vi "CLD 16 solution.vi"() -> ()   [LabVIEW 2020]
doc: "CLD 16 Exercise"
uses:
  Controls/CLD 16 Control Panel.ctl
  Controls/CLD 16 Status Panel.ctl
panel:
  in  "Stop Button":bool
  out "Line Two Active":bool
  out "Line One Active":bool
  in  "Control Panel Two":T1 {"Tons of Peanuts" scale=0.0..10.0}
  out "Process Control":T2 {"Process Value" format="%#.3g"}
  in  "Control Panel One":T1 {"Tons of Peanuts" scale=0.0..10.0}
  # "Display Panel"
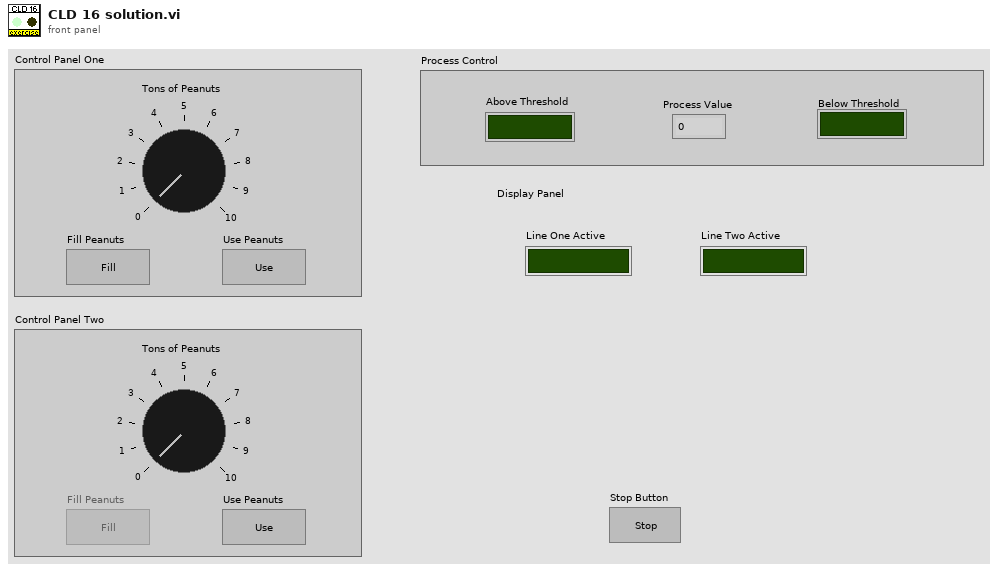
[diagram p1: front panel]
types:
  T1 = typedef "CLD 16 Control Panel.ctl" = cluster{"Tons of Peanuts":i8, "Fill Peanuts":bool, "Use Peanuts":bool}
  T2 = typedef "CLD 16 Status Panel.ctl" = cluster{"Above Threshold":bool, "Below Threshold":bool, "Process Value":dbl}
  T3 = enum8{"Enabled", "Disabled", "Disabled and Grayed Out"}
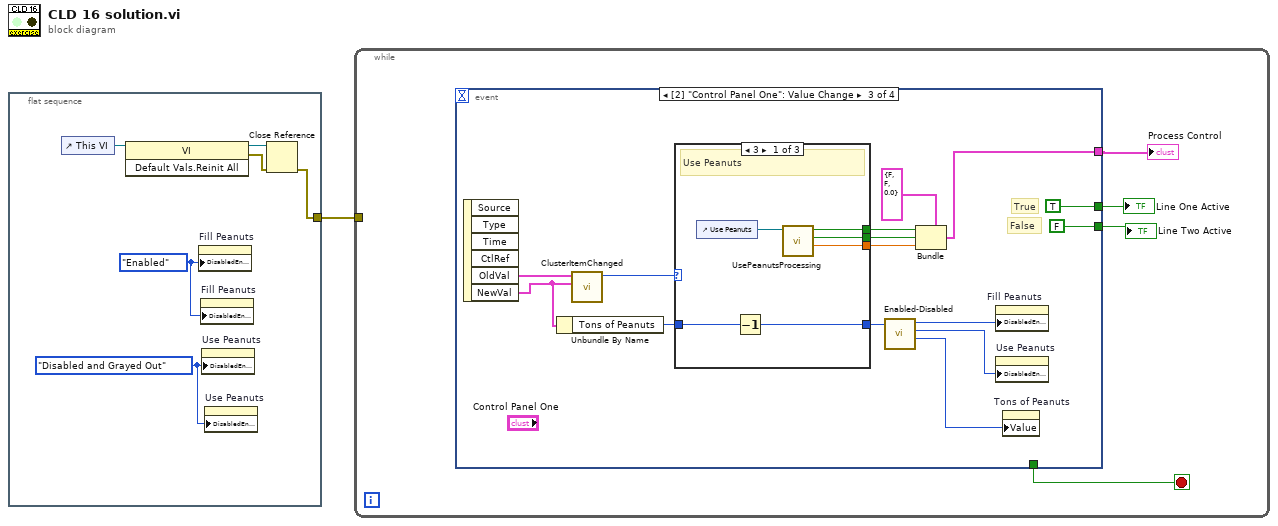
[diagram p0: block diagram]
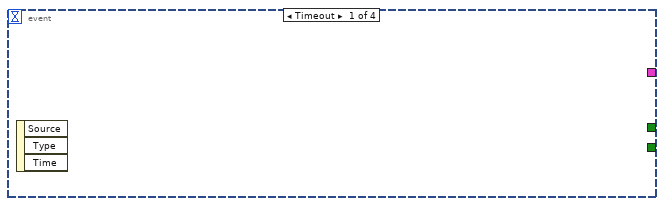
[diagram p2: hidden frame]
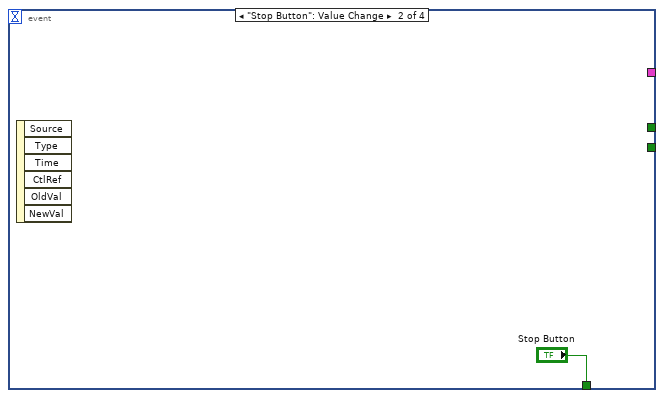
[diagram p3: hidden frame]
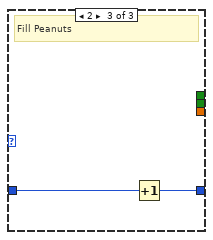
[diagram p5: hidden frame]
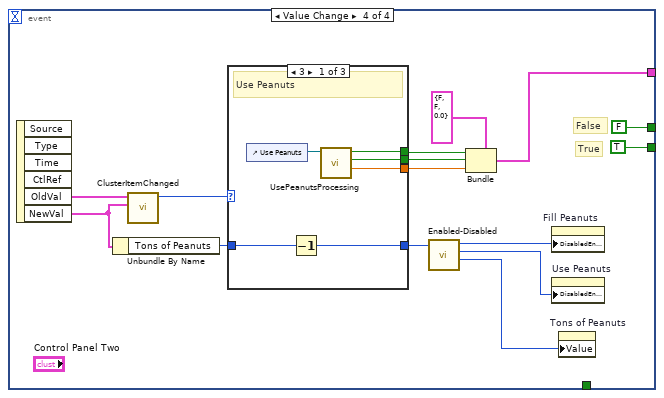
[diagram p6: hidden frame]
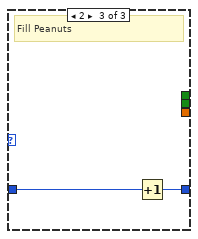
[diagram p8: hidden frame]
diagram:
  n1 = flat-sequence {
    tunnel: [w4] -> w1
    frame #0 {
      w2 = T3."Disabled and Grayed Out" ("Disabled")
      w3 = T3."Enabled" ("Disabled")
      n2 = control-ref of="This VI"() -> (w5:refnum<vi>)
      n3 = invoke class="VI" method="Default Vals.Reinit All"(reference=w5) -> (reference out=w6:refnum<vi>, error out=w7:errorcluster)  [unwired: 2 in, 1 out]
      n4 = property on="Fill Peanuts" class="Bool"("DisabledEnum"=w3) -> ()  [unwired: 2 in, 2 out]
      n5 = property on="Fill Peanuts" class="Bool"("DisabledEnum"=w3) -> ()  [unwired: 2 in, 2 out]
      n6 = property on="Use Peanuts" class="Bool"("DisabledEnum"=w2) -> ()  [unwired: 2 in, 2 out]
      n7 = property on="Use Peanuts" class="Bool"("DisabledEnum"=w2) -> ()  [unwired: 2 in, 2 out]
      n8 = Close Reference(reference=w6, error in (no error)=w7) -> (error out=w4:errorcluster)
    }
  }
  n9 = while {
    tunnel: w1 -> [_]
    stop <- w11 stop-if-true
    n10 = event shown="[2] \"Control Panel One\": Value Change" {
      selector: _ -> [_ _ _ _]
      dyn-events: _ -> [_ _ _ _]
      timeout: _ -> [_ _ _ _]
      tunnel: [_ "Stop Button" _ _] -> w11
      tunnel: [_ _ FALSE ("Line Two Active") TRUE ("Line Two Active")] -> w10
      tunnel: [_ _ TRUE ("Line One Active") FALSE ("Line One Active")] -> w9
      tunnel: [_ _ w13 w37] -> w8
      event Timeout {
        n11 = event-data() -> ()  [unwired: 1 in, 3 out]
      }
      event "Stop Button": Value Change {
        n12 = event-data() -> ()  [unwired: 1 in, 6 out]
      }
      event Value Change {
        # "False"
        # "True"
        n13 = event-data() -> ("OldVal"=w27:T1, "NewVal"=w23:T1)  [unwired: 1 in, 4 out]
        n14 = Unbundle By Name(w23) -> ("Tons of Peanuts"=w22:i8)
        n15 = call "ClusterItemChanged.vi"("NewVal"=w23, "OldVal"=w27) -> ("Numeric"=w26:i32)  [unwired: 9 in]
        n16 = case shown="3" w26 {
          tunnel: w22 -> [w33 w34 w36]
          tunnel: [w32 w34 w35] -> w21
          tunnel: [w30 _ _] -> w16
          tunnel: [w29 _ _] -> w15
          tunnel: [w28 _ _] -> w14
          frame 3 {
            # "Use Peanuts"
            n17 = control-ref of="Use Peanuts"() -> (w31:refnum<vi>)
            n18 = Decrement(x=w33) -> (x-1=w32:i8)
            n19 = call "UsePeanutsProcessing.vi"("Boolean in"=w31) -> ("Process Value"=w28:dbl, "Below Threshold"=w29:bool, "Above Threshold"=w30:bool)  [unwired: 8 in]
          }
          frame 1, Default {
            # "Tons of Peanuts"
          }
          frame 2 {
            # "Fill Peanuts"
            n20 = Increment(x=w36) -> (x+1=w35:i8)
          }
        }
        n21 = call "Enabled-Disabled.vi"("Tons of Peanuts"=w21) -> ("Tons of Peanuts"=w20:i8, "Use Peanuts Control Status"=w24:T3, "Fill Peanuts Control Status"=w25:T3)  [unwired: 8 in]
        n22 = Bundle(cluster=T2 {"Above Threshold"=FALSE, "Below Threshold"=FALSE, "Process Value"=0.0} ("Process Control"), "Above Threshold"=w16, "Below Threshold"=w15, "Process Value"=w14) -> (w13:T2)
        n23 = property on="Fill Peanuts" class="Bool"("DisabledEnum"=w25) -> ()  [unwired: 2 in, 2 out]
        n24 = property on="Use Peanuts" class="Bool"("DisabledEnum"=w24) -> ()  [unwired: 2 in, 2 out]
        n25 = property on="Tons of Peanuts" class="Knob (strict)"("Value"=w20) -> ()  [unwired: 2 in, 2 out]
      }
      event Value Change {
        # "False"
        # "True"
        n26 = event-data() -> ("OldVal"=w42:T1, "NewVal"=w43:T1)  [unwired: 1 in, 4 out]
        n27 = Unbundle By Name(w43) -> ("Tons of Peanuts"=w48:i8)
        n28 = call "ClusterItemChanged.vi"("NewVal"=w43, "OldVal"=w42) -> ("Numeric"=w51:i32)  [unwired: 9 in]
        n29 = case shown="3" w51 {
          tunnel: w48 -> [w57 w58 w60]
          tunnel: [w56 w58 w59] -> w47
          tunnel: [w55 _ _] -> w40
          tunnel: [w54 _ _] -> w39
          tunnel: [w53 _ _] -> w38
          frame 3 {
            # "Use Peanuts"
            n30 = control-ref of="Use Peanuts"() -> (w52:refnum<vi>)
            n31 = Decrement(x=w57) -> (x-1=w56:i8)
            n32 = call "UsePeanutsProcessing.vi"("Boolean in"=w52) -> ("Process Value"=w53:dbl, "Below Threshold"=w54:bool, "Above Threshold"=w55:bool)  [unwired: 8 in]
          }
          frame 1, Default {
            # "Tons of Peanuts"
          }
          frame 2 {
            # "Fill Peanuts"
            n33 = Increment(x=w60) -> (x+1=w59:i8)
          }
        }
        n34 = call "Enabled-Disabled.vi"("Tons of Peanuts"=w47) -> ("Tons of Peanuts"=w46:i8, "Use Peanuts Control Status"=w49:T3, "Fill Peanuts Control Status"=w50:T3)  [unwired: 8 in]
        n35 = Bundle(cluster=T2 {"Above Threshold"=FALSE, "Below Threshold"=FALSE, "Process Value"=0.0} ("Process Control"), "Above Threshold"=w40, "Below Threshold"=w39, "Process Value"=w38) -> (w37:T2)
        n36 = property on="Fill Peanuts" class="Bool"("DisabledEnum"=w50) -> ()  [unwired: 2 in, 2 out]
        n37 = property on="Use Peanuts" class="Bool"("DisabledEnum"=w49) -> ()  [unwired: 2 in, 2 out]
        n38 = property on="Tons of Peanuts" class="Knob (strict)"("Value"=w46) -> ()  [unwired: 2 in, 2 out]
      }
    }
    "Line Two Active" <- w10
    "Line One Active" <- w9
    "Process Control" <- w8
  }
